vi "FeedbackDecode_BuildMSMSPacket.vi"(1 "Value":sgl[](array[numeric]), 2 "FNum":i16, 3 "CompIdx":i32, 4 "CompArray":T1(array[cluster])) -> (0 "CompPacket":i8[](array[numeric]))   [LabVIEW 2020]
panel:
  out "N":i8[](array[numeric])
  out "ID":i8[](array[numeric])
  out "FN":i8[](array[numeric])
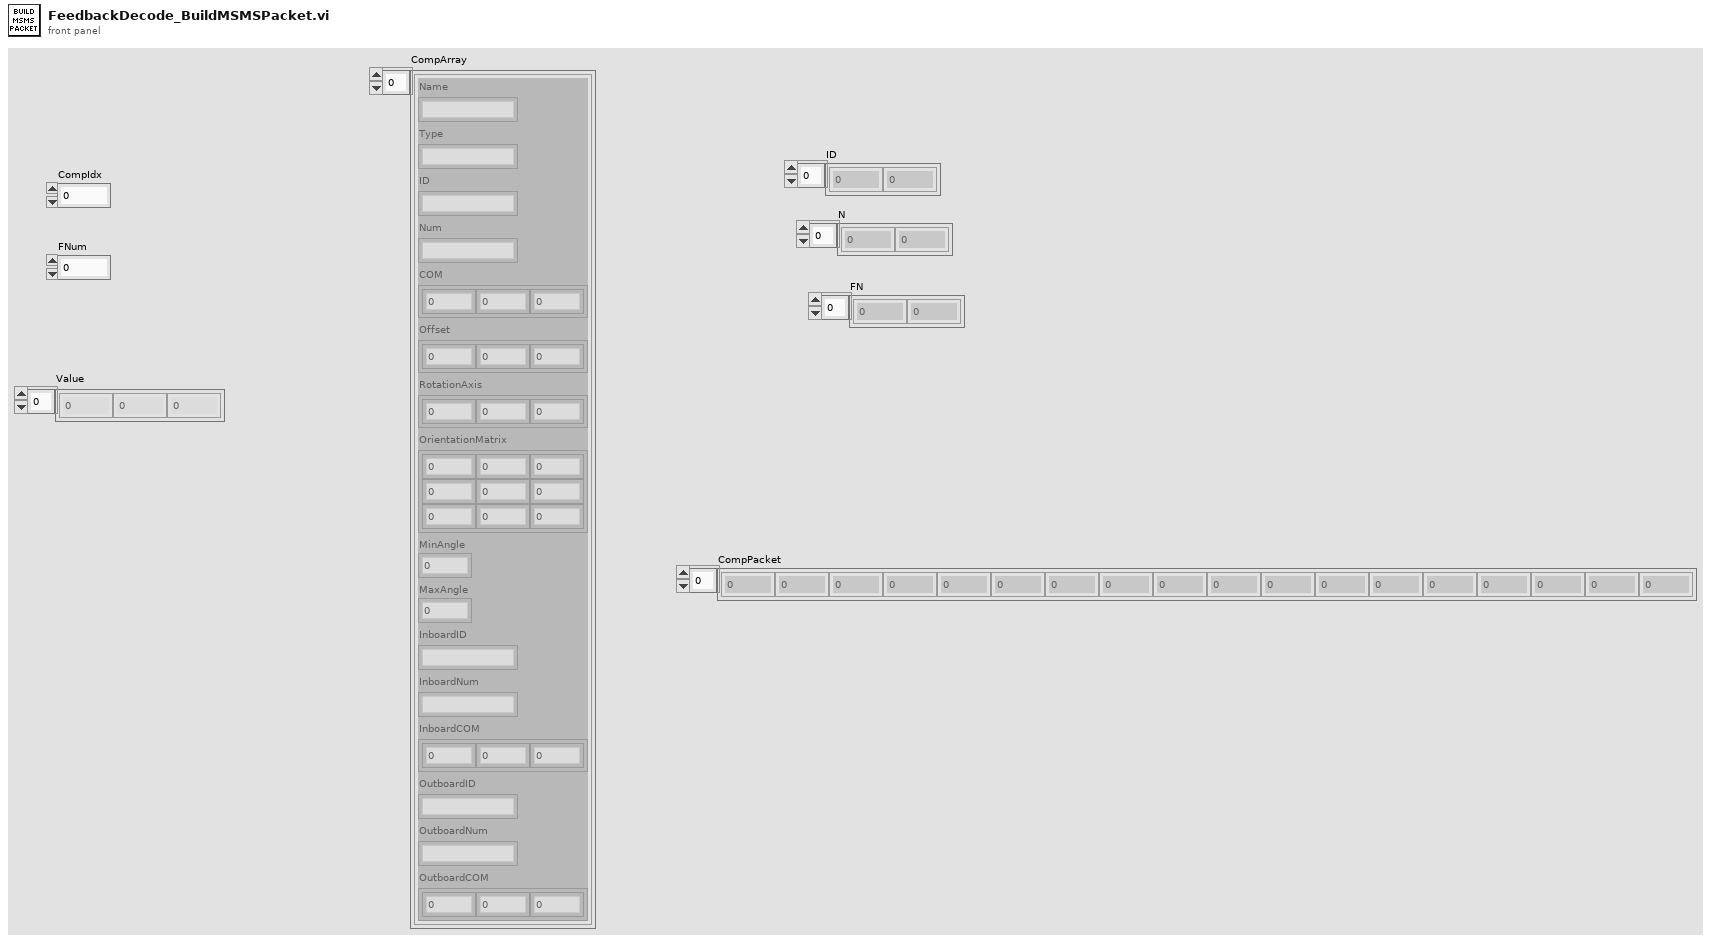
[diagram p1: front panel]
types:
  T1 = cluster{"Name":string, "Type":string, "ID":string, "Num":string, "COM":dbl[], "Offset":dbl[], "RotationAxis":dbl[], "OrientationMatrix":dbl[][], "MinAngle":dbl, "MaxAngle":dbl, "InboardID":string, "InboardNum":string, "InboardCOM":dbl[], "OutboardID":string, "OutboardNum":string, "OutboardCOM":dbl[]}[]
  T2 = cluster{"Name":string, "Type":string, "ID":string, "Num":string, "COM":dbl[], "Offset":dbl[], "RotationAxis":dbl[], "OrientationMatrix":dbl[][], "MinAngle":dbl, "MaxAngle":dbl, "InboardID":string, "InboardNum":string, "InboardCOM":dbl[], "OutboardID":string, "OutboardNum":string, "OutboardCOM":dbl[]}
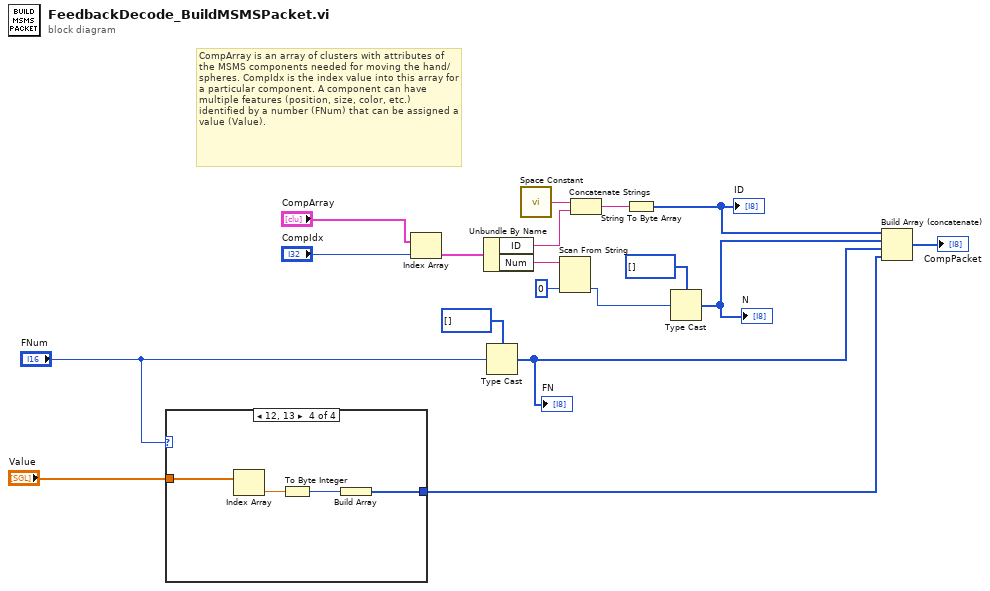
[diagram p0: block diagram]
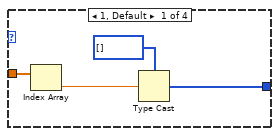
[diagram p2: hidden frame]
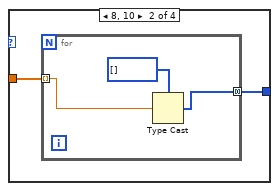
[diagram p3: hidden frame]
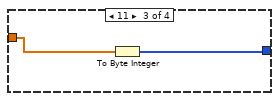
[diagram p4: hidden frame]
diagram:
  # "CompArray is an array of clusters with attributes of the MSMS components needed for moving the hand/spheres. CompIdx is the index value into this array for a particular component. A component can have multiple features (position, size, color, etc.) identified by a number (FNum) that can be assigned a value (Value)."
  n1 = case shown="12, 13" "FNum" {
    tunnel: [w21 w23 w28 w30] -> w5
    tunnel: "Value" -> [w20 w24 w29 w33]
    frame 1, Default {
      n2 = Index Array(array=w20) -> (element=w19:sgl)  [unwired: 1 in]
      n3 = Type Cast(type=i8[] [], x=w19) -> (*(type *) &x=w21:i8[])
    }
    frame 8, 10 {
      n4 = for {
        tunnel: w24 -> [w26] mode=indexing
        tunnel: [w25] -> w23 mode=concatenating
        n5 = Type Cast(type=i8[] [], x=w26) -> (*(type *) &x=w25:i8[])
      }
    }
    frame 11 {
      n6 = To Byte Integer(number=w29) -> (8bit integer=w28:i8[])
    }
    frame 12, 13 {
      n7 = Index Array(array=w33) -> (element=w32:sgl)  [unwired: 1 in]
      n8 = To Byte Integer(number=w32) -> (8bit integer=w31:i8)
      n9 = Build Array(w31) -> (w30:i8[])
    }
  }
  n10 = Index Array(array="CompArray", index="CompIdx") -> (element=w17:T2)
  n11 = Unbundle By Name(w17) -> ("ID"=w16:string, "Num"=w12:string)
  n12 = Type Cast(type=i8[] [], x="FNum") -> (*(type *) &x=w6:i8[])
  "FN" <- w6
  n13 = call <vilib>:"Space Constant.vi"() -> ("String"=w15:string)
  n14 = Scan From String(input string=w12, default 1=i16 0) -> (output 1=w10:i16)  [unwired: 3 in, 3 out]
  n15 = Concatenate Strings(w15, w16) -> (w14:string)
  n16 = String To Byte Array(string=w14) -> (unsigned byte array=w8:u8[])
  "ID" <- w8
  n17 = Type Cast(type=i8[] [], x=w10) -> (*(type *) &x=w7:i8[])
  "N" <- w7
  n18 = Build Array (concatenate)(w8, w7, w6, w5) -> (→"CompPacket":u8[])
